vi "Hacking FFID header info in raw data files.vi"(8 "New Bkgnd Variance":string[](array[string]), 9 "New Bkgnd Values":string[](array[string]), 10 "Time":string, 11 "file (use dialog)":path) -> ()   [LabVIEW 2022 SP3]
panel:
  out "Fianl subarray":string[](array[string])
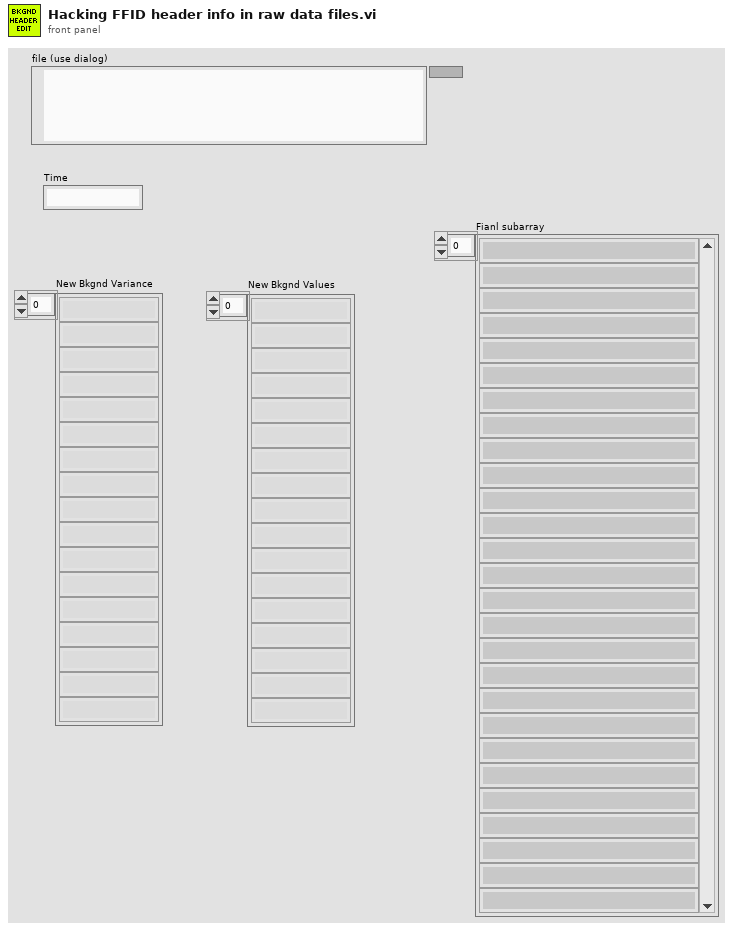
[diagram p1: front panel]
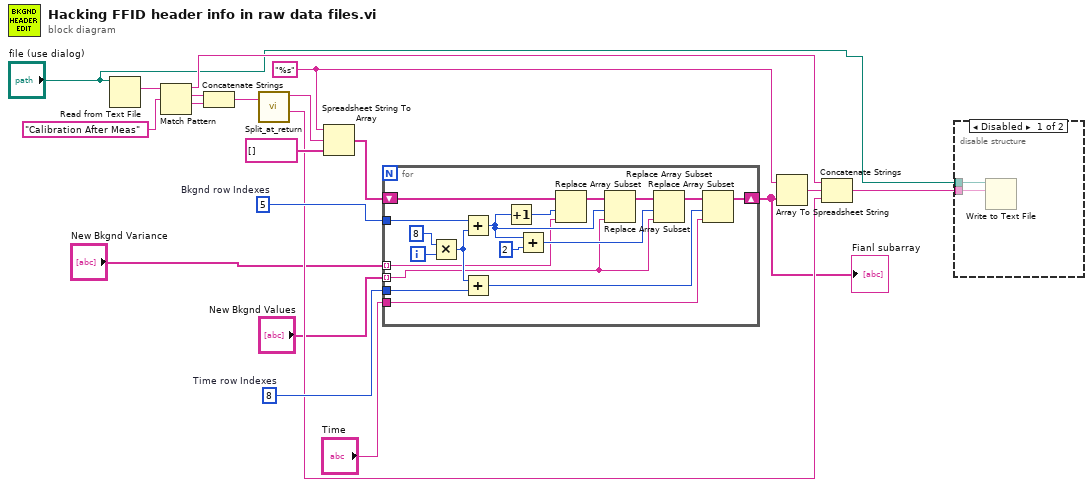
[diagram p0: block diagram]
diagram:
  w11 = "%s" ("format string")
  w19 = 8  # Time row Indexes
  w20 = 5  # Bkgnd row Indexes
  n1 = Read from Text File(file (use dialog)="file (use dialog)") -> (text=w17:string)  [unwired: 3 in, 3 out]
  n2 = Match Pattern(string=w17, regular expression="Calibration After Meas") -> (before substring=w10:string, match substring=w16:string, after substring=w15:string)  [unwired: 1 in, 1 out]
  n3 = Concatenate Strings(w16, w15) -> (w14:string)
  n4 = call "Split_at_return.vi"("String"=w14) -> ("before substring"=w13:string, "after substring"=w8:string)  [unwired: 1 in, 2 out]
  n5 = Spreadsheet String To Array(format string=w11, spreadsheet string=w13, array type (2D Dbl)=string[] []) -> (array=w6:string[])  [unwired: 1 in]
  n6 = for {
    tunnel: w20 -> [w38]
    tunnel: w19 -> [w34]
    shift-right: [w28] -> w5
    shift-left: w6 -> [w25]
    tunnel: "New Bkgnd Values" -> [w27] mode=indexing
    tunnel: "Time" -> [w26]
    tunnel: "New Bkgnd Variance" -> [w21] mode=indexing
    i -> [w35]
    n7 = Multiply(x=8 ("y"), y=w35) -> (x*y=w33:i32)
    n8 = Add(x=w38, y=w33) -> (x+y=w23:i32)
    n9 = Add(x=w33, y=w34) -> (x+y=w31:i32)
    n10 = Increment(x=w23) -> (x+1=w22:i32)
    n11 = Add(x=w23, y=2) -> (x+y=w32:i32)
    n12 = Replace Array Subset(array=w25, new element=w21, index=w22) -> (w24:string[])
    n13 = Replace Array Subset(array=w24, new element=w27, index=w23) -> (w30:string[])
    n14 = Replace Array Subset(array=w30, new element=w27, index=w32) -> (w29:string[])
    n15 = Replace Array Subset(array=w29, new element=w26, index=w31) -> (w28:string[])
  }
  "Fianl subarray" <- w5
  n16 = Array To Spreadsheet String(array=w5, 3:w11) -> (spreadsheet string=w9:string)  [unwired: 1 in]
  n17 = Concatenate Strings(w10, w9, w8) -> (w7:string)
  n18 = disable-structure shown="Disabled" {
    disable-tunnel: w7 -> [w40 _]
    disable-tunnel: "file (use dialog)" -> [w39 _]
    frame Disabled {
      n19 = Write to Text File(file (use dialog)=w39, text=w40) -> ()  [unwired: 2 in, 3 out]
    }
    frame Enabled {
    }
  }
